vi "cmdEdit.vi"(8 "error in (no error)":errorcluster, 11 "connection ID":refnum<k5>) -> (0 "error out":errorcluster, 2 "Command":string, 3 "connection ID out":refnum<k5>)   [LabVIEW 2010]
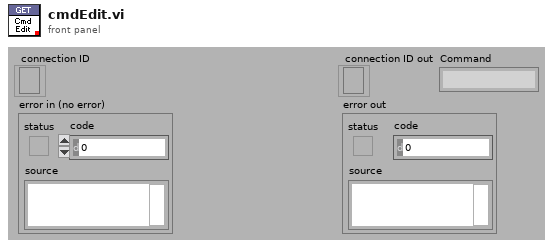
[diagram p1: front panel]
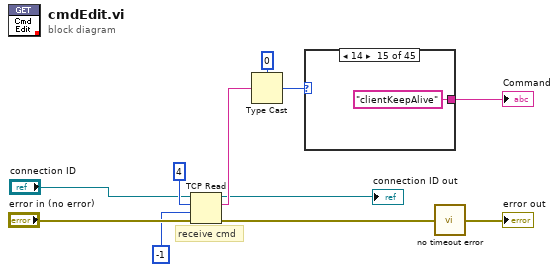
[diagram p0: block diagram]
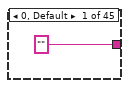
[diagram p2: hidden frame]
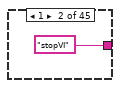
[diagram p3: hidden frame]
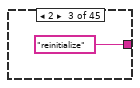
[diagram p4: hidden frame]
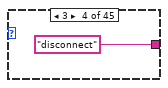
[diagram p5: hidden frame]
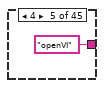
[diagram p6: hidden frame]
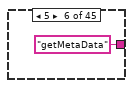
[diagram p7: hidden frame]
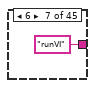
[diagram p8: hidden frame]
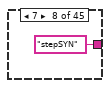
[diagram p9: hidden frame]
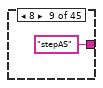
[diagram p10: hidden frame]
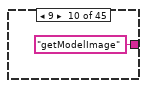
[diagram p11: hidden frame]
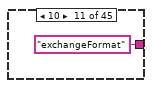
[diagram p12: hidden frame]
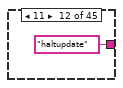
[diagram p13: hidden frame]
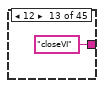
[diagram p14: hidden frame]
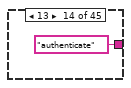
[diagram p15: hidden frame]
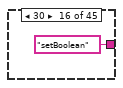
[diagram p16: hidden frame]
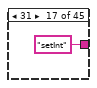
[diagram p17: hidden frame]
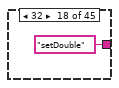
[diagram p18: hidden frame]
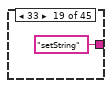
[diagram p19: hidden frame]
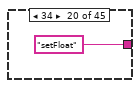
[diagram p20: hidden frame]
diagram:
  # "receive cmd"
  n1 = TCP Read(connection ID="connection ID", bytes to read=4, error in (no error)="error in (no error)", 9:-1 ("timeout ms (25000)")) -> (connection ID out=→"connection ID out":refnum<k5>, data out=w10:string, error out=w3:errorcluster)  [unwired: 1 out]
  n2 = Type Cast(type=0, x=w10) -> (*(type *) &x=w5:i32)
  n3 = case shown="14" w5 {
    tunnel: ["" "stopVI" "reinitialize" "disconnect" "openVI" "getMetaData" "runVI" "stepSYN" "stepAS" "getModelImage" "exchangeFormat" "haltupdate" "closeVI" "authenticate" "clientKeepAlive" "setBoolean" "setInt" "setDouble" "setString" "setFloat" "setBooleanArray" "setIntArray" "setDoubleArray" "setStringArray" "setFloatArray" "setBooleanArray2D" "setIntArray2D" "setDoubleArray2D" "setStringArray2D" "setFloatArray2D" "getBoolean" "getInt" "getDouble" "getString" "getFloat" "getBooleanArray" "getIntArray" "getDoubleArray" "getStringArray" "getFloatArray" "getBooleanArray2D" "getIntArray2D" "getDoubleArray2D" "getStringArray2D" "getFloatArray2D"] -> w4
    frame 0, Default {
    }
    frame 1 {
    }
    frame 2 {
    }
    frame 3 {
    }
    frame 4 {
    }
    frame 5 {
    }
    frame 6 {
    }
    frame 7 {
    }
    frame 8 {
    }
    frame 9 {
    }
    frame 10 {
    }
    frame 11 {
    }
    frame 12 {
    }
    frame 13 {
    }
    frame 14 {
    }
    frame 30 {
    }
    frame 31 {
    }
    frame 32 {
    }
    frame 33 {
    }
    frame 34 {
    }
    frame 40 {
    }
    frame 41 {
    }
    frame 42 {
    }
    frame 43 {
    }
    frame 44 {
    }
    frame 50 {
    }
    frame 51 {
    }
    frame 52 {
    }
    frame 53 {
    }
    frame 54 {
    }
    frame 60 {
    }
    frame 61 {
    }
    frame 62 {
    }
    frame 63 {
    }
    frame 64 {
    }
    frame 70 {
    }
    frame 71 {
    }
    frame 72 {
    }
    frame 73 {
    }
    frame 74 {
    }
    frame 80 {
    }
    frame 81 {
    }
    frame 82 {
    }
    frame 83 {
    }
    frame 84 {
    }
  }
  "Command" <- w4
  n4 = call "no timeout error.vi"("error in (no error)"=w3) -> ("error out"=→"error out":errorcluster)
